vi "Zero.vi"(8 "error in (no error)":errorcluster, 10 "Channel (1: Channel A)":u16(ring)=1 items=["Channel A"=1, "Channel B"=2], 11 "VISA resource name":refnum<visa-resource-name>) -> (0 "error out":errorcluster, 3 "VISA resource name out":refnum<visa-resource-name>)   [LabVIEW 2020, in "Template - Power Meter.lvlib"]
doc: "Performs a zero correction on the specified channel."
uses:
  <instrlib>/_Template - Power Meter/Template - Power Meter.lvlib
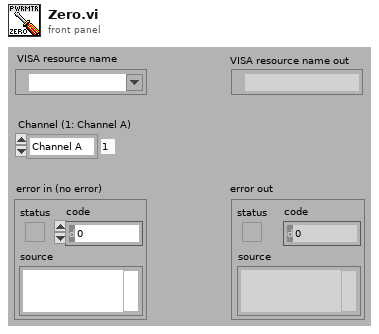
[diagram p1: front panel]
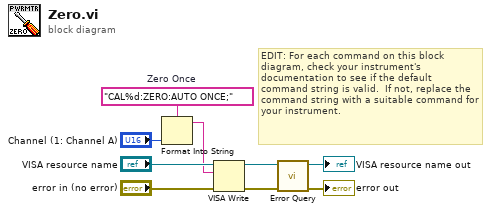
[diagram p0: block diagram]
diagram:
  w8 = "CAL%d:ZERO:AUTO ONCE;"  # Zero Once
  # "EDIT: For each command on this block diagram, check your instrument's documentation to see if the default command string is valid.  If not, replace the command string with a suitable command for your instrument."
  n1 = Format Into String(format string=w8, "Channel (1: Channel A)") -> (resulting string=w1:string)  [unwired: 2 in, 1 out]
  n2 = VISA Write(VISA resource name="VISA resource name", write buffer=w1, error in (no error)="error in (no error)") -> (VISA resource name out=w5:refnum<visa-resource-name>, error out=w3:errorcluster)  [unwired: 1 out]
  n3 = call <instrlib>:"Error Query.vi"("error in (no error)"=w3, "VISA resource name"=w5) -> ("error out"=→"error out":errorcluster, "VISA resource name out"=→"VISA resource name out":refnum<visa-resource-name>)  [unwired: 6 in, 2 out]
